vi "Tach Process Digital (1 Ch).vi"(0 "digital pulses":dbl[](array[numeric]), 3 "pulse/revolution (1)":i32=1, 4 "OS Clk Start":dbl, 8 "Empty Block Cutoff":i32, 9 "tach state in":T1) -> (13 "tach state out":T1, 14 "speed position info":T3, 18 "Instant RPM":dbl)   [LabVIEW 2017, in "VibrationAnalysisFunctions.lvlib"]
uses:
  <vilib>/addons/InsightCM/Utilities/Analysis/Vibration/VibrationAnalysisFunctions.lvlib
  <vilib>/addons/Sound and Vibration/Order Analysis/Misc/OAT Position Info.ctl
  <vilib>/addons/InsightCM/Utilities/Analysis/Vibration/controls/Tachometer.ctl
  <vilib>/addons/InsightCM/Utilities/Analysis/Vibration/controls/DigitalTachometer.ctl
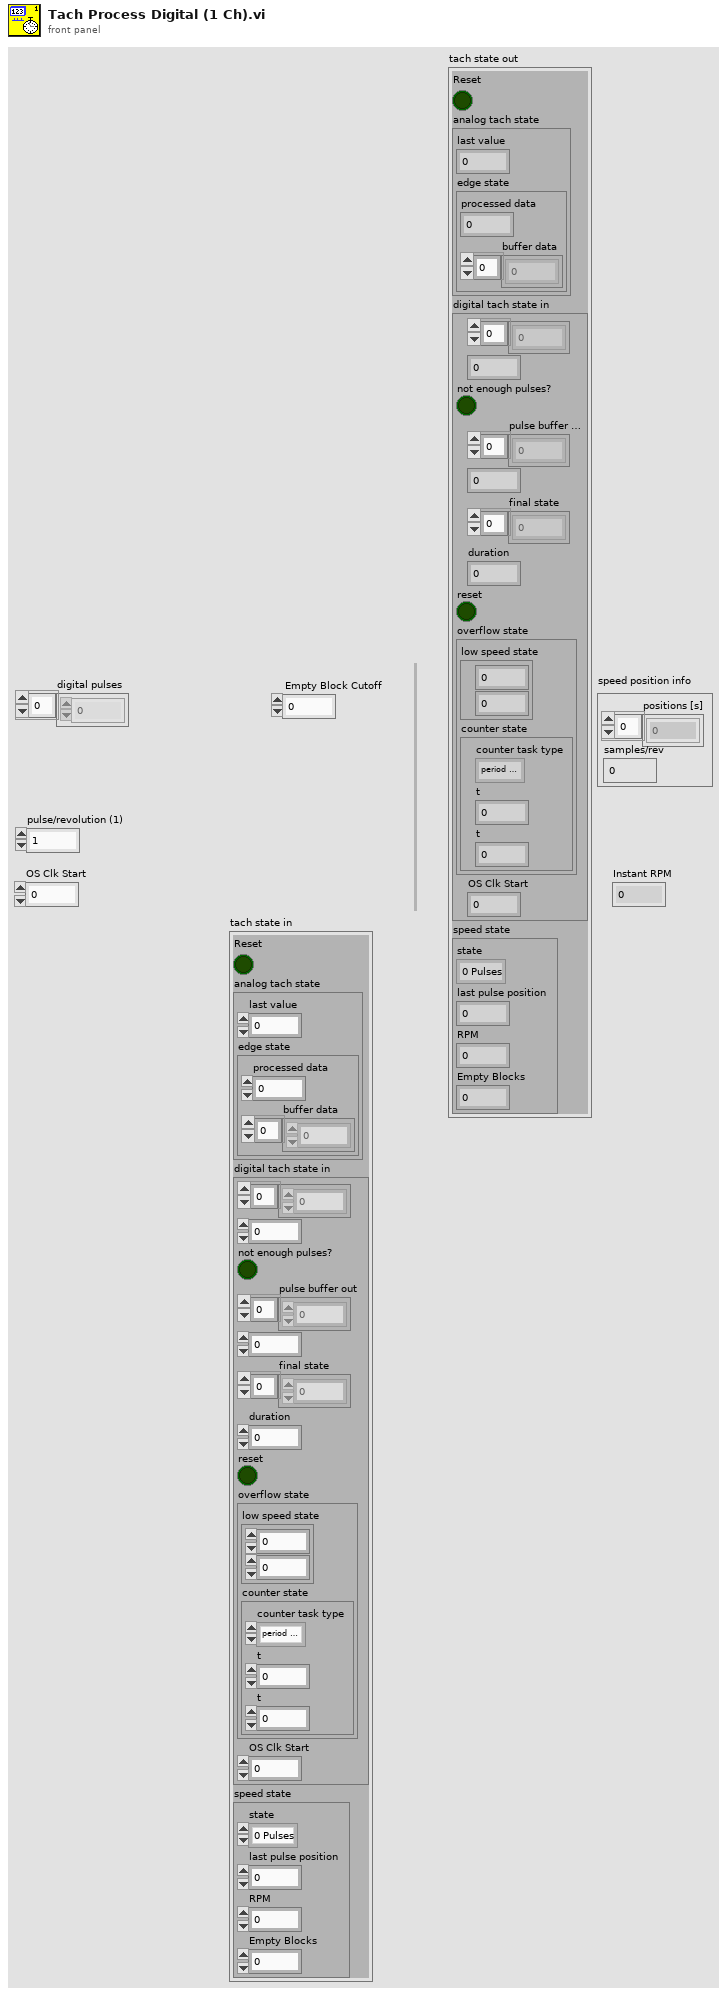
[diagram p1: front panel]
types:
  T1 = typedef "VibrationAnalysisFunctions.lvlib/Tachometer.ctl" = cluster{"Reset":bool, "analog tach state":cluster{"last value":dbl, "edge state":cluster{"processed data":dbl, "buffer data":dbl[]}}, "digital tach state in":T2, "speed state":cluster{"state":enum16{"0 Pulses", "1 Pulse", "2+ Pulses"}, "last pulse position":dbl, "RPM":dbl, "Empty Blocks":i32}}
  T2 = typedef "VibrationAnalysisFunctions.lvlib/DigitalTachometer.ctl" = cluster{dbl[], i32, "not enough pulses?":bool, "pulse buffer out":dbl[], i32, "final state":dbl[], "duration":dbl, "reset":bool, "overflow state":cluster{"low speed state":cluster{dbl, ext}, "counter state":cluster{"counter task type":enum16{"period measurement", "event counting"}, "t":dbl, "t":dbl}}, "OS Clk Start":dbl}
  T3 = typedef "OAT Position Info.ctl" = cluster{"positions [s]":dbl[], "samples/rev":dbl}
  T4 = cluster{"state":enum16{"0 Pulses", "1 Pulse", "2+ Pulses"}, "last pulse position":dbl, "RPM":dbl, "Empty Blocks":i32}
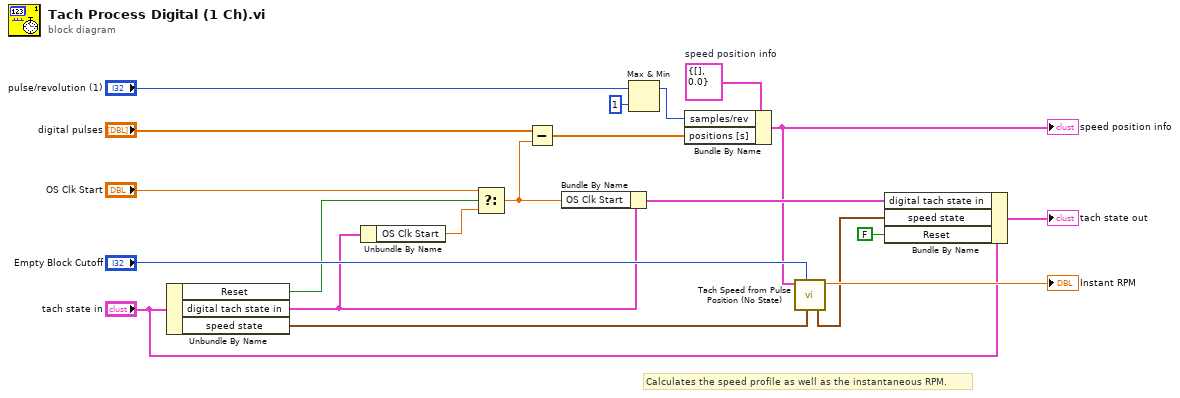
[diagram p0: block diagram]
diagram:
  w3 = T3 {"positions [s]"=[], "samples/rev"=0.0}  # speed position info
  # "Calculates the speed profile as well as the instantaneous RPM."
  n1 = Unbundle By Name("tach state in") -> ("Reset"=w12:bool, "digital tach state in"=w2:T2, "speed state"=w16:T4)
  n2 = Unbundle By Name(w2) -> ("OS Clk Start"=w9:dbl)
  n3 = Select(t="OS Clk Start", s=w12, f=w9) -> (s? t:f=w8:dbl)
  n4 = Subtract(x="digital pulses", y=w8) -> (x-y=w1:dbl[])
  n5 = Bundle By Name(cluster=w2, "OS Clk Start"=w8) -> (w13:T2)
  n6 = Max & Min(x="pulse/revolution (1)", y=1) -> (max(x,y)=w4:i32)  [unwired: 1 out]
  n7 = Bundle By Name(cluster=w3, "samples/rev"=w4, "positions [s]"=w1) -> (w7:T3)
  "speed position info" <- w7
  n8 = call <vilib>:"Tach Speed from Pulse Position (No State).vi"("state in"=w16, "Empty Block Cutoff"="Empty Block Cutoff", "speed position info"=w7) -> ("RPM"=→"Instant RPM":dbl, "state out"=w18:T4)  [unwired: 7 in]
  n9 = Bundle By Name(cluster="tach state in", "digital tach state in"=w13, "speed state"=w18, "Reset"=FALSE) -> (→"tach state out":T1)
